vi "Bode Magnitude Plot.vi"() -> ()   [LabVIEW 2015]
uses:
  <vilib>/Analysis/NI_AALPro.lvlib
panel:
  out "XY Graph":cluster{dbl[], dbl[]}(graph)
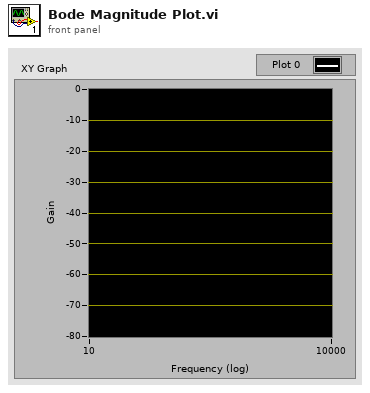
[diagram p1: front panel]
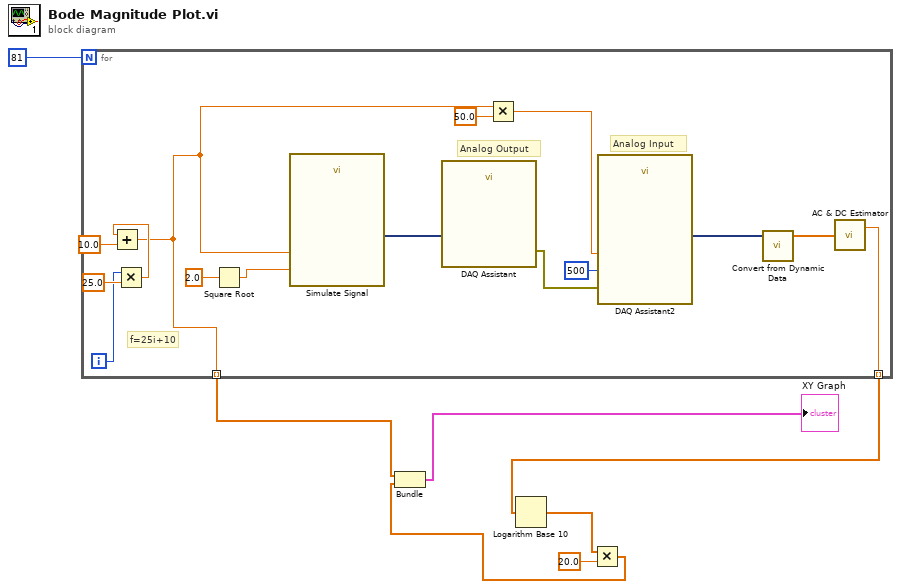
[diagram p0: block diagram]
diagram:
  n1 = for {
    N: 81 -> [_]
    tunnel: [w9] -> w3 mode=indexing
    tunnel: [w8] -> w6 mode=indexing
    i -> [w11]
    # "f=25i+10"
    # "Analog Input"
    # "Analog Output"
    n2 = Multiply(x=w11, y=25.0) -> (x*y=w10:dbl)
    n3 = Add(x=w10, y=10.0) -> (x+y=w9:dbl)
    n4 = Square Root(x=2.0) -> (sqrt(x)=w21:dbl)
    n5 = call "Simulate Signal"("Frequency"=w9, "Amplitude"=w21) -> ("Sine"=w20:dynamicdata)  [unwired: 12 in, 1 out]
    n6 = call "DAQ Assistant"("data"=w20) -> ("error out"=w19:errorcluster)  [unwired: 17 in, 1 out]
    n7 = Multiply(x=w9, y=50.0) -> (x*y=w17:dbl)
    n8 = call "DAQ Assistant2"("rate"=w17, "number of samples"=500, "error in"=w19) -> ("data"=w15:dynamicdata)  [unwired: 13 in, 3 out]
    n9 = call "Convert from Dynamic Data"("Dynamic Data Type"=w15) -> ("Array"=w14:dbl[])  [unwired: 3 in]
    n10 = call <vilib>:"AC & DC Estimator.vi"("Signal (V)"=w14) -> ("AC estimate (Vrms)"=w8:dbl)  [unwired: 1 out]
  }
  n11 = Logarithm Base 10(1:w6) -> (0:w4:dbl[])
  n12 = Multiply(x=w4, y=20.0) -> (x*y=w2:dbl[])
  n13 = Bundle(w3, w2) -> (→"XY Graph":cluster{dbl[], dbl[]})  [unwired: 1 in]
